vi "Add Menu Items.vi"(7 "Menu control":enum16{"Pulse", "Post-process", "Monitor"}(ring), 8 "error in (no error)":errorcluster, 9 "Reset":bool, 10 "Item Names":string[](array[string]), 11 "Monitor-Pulse in":refnum<class "Application Controller.lvclass">) -> (0 "error out":errorcluster, 3 "Monitor-Pulse out":refnum<class "Application Controller.lvclass">)   [LabVIEW 2016, in "Application Controller.lvclass"]
uses:
  Application Controller.lvclass
  Application Controller.lvclass/Application Controller.ctl
  Read Monitor ref.vi
  Write Monitor ref.vi
  Read Postproc ref.vi
  Write Postproc ref.vi
  NHMFL_Core/Libraries/Queued Listbox/Queued Listbox.xctl
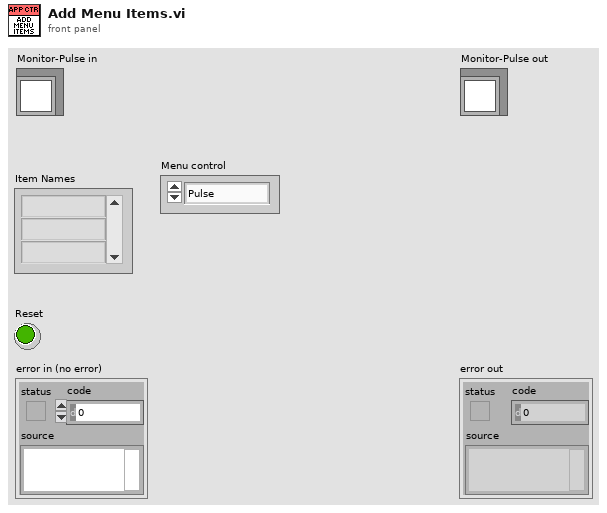
[diagram p1: front panel]
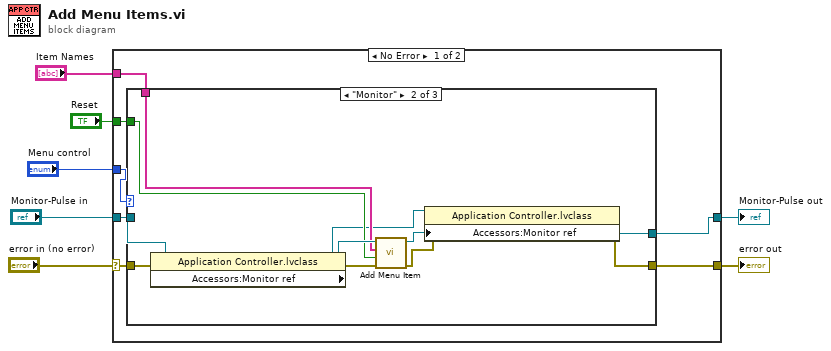
[diagram p0: block diagram]
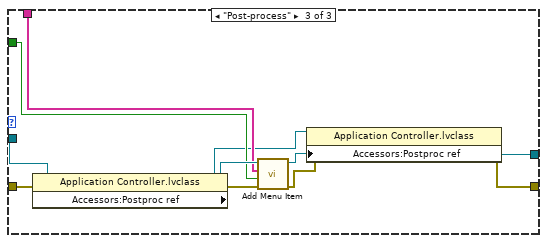
[diagram p3: hidden frame]
diagram:
  n1 = case shown="No Error" "error in (no error)" {
    selector: "error in (no error)" -> [w10 w40]
    tunnel: [w9 w40] -> w6
    tunnel: [w14 w39] -> w4
    tunnel: "Monitor-Pulse in" -> [w11 w39]
    tunnel: "Item Names" -> [w13 _]
    tunnel: "Reset" -> [w12 _]
    tunnel: "Menu control" -> [w8 _]
    frame No Error {
      n2 = case shown="\"Monitor\"" w8 {
        tunnel: [w16 w25 w36] -> w14
        tunnel: w13 -> [_ w24 w35]
        tunnel: w12 -> [_ w23 w34]
        tunnel: w11 -> [w16 w22 w33]
        tunnel: w10 -> [w15 w19 w30]
        tunnel: [w15 w18 w29] -> w9
        frame "Pulse", Default {
        }
        frame "Monitor" {
          n3 = property class="Application Controller.lvclass"(reference=w22, error in=w19) -> (reference out=w21:refnum<class "Application Controller.lvclass">, error out=w20:errorcluster, "Accessors:Monitor ref"=w27:refnum<vi>)
          n4 = call "Add Menu Item.vi"("error in (no error)"=w20, "Reset"=w23, "Item Names"=w24, "Queed Listbox ref"=w27) -> ("error out"=w17:errorcluster, "Queed Listbox ref out"=w26:refnum<vi>)  [unwired: 5 in, 1 out]
          n5 = property class="Application Controller.lvclass"(reference=w21, error in=w17, "Accessors:Monitor ref"=w26) -> (reference out=w25:refnum<class "Application Controller.lvclass">, error out=w18:errorcluster)
        }
        frame "Post-process" {
          n6 = property class="Application Controller.lvclass"(reference=w33, error in=w30) -> (reference out=w32:refnum<class "Application Controller.lvclass">, error out=w31:errorcluster, "Accessors:Postproc ref"=w38:refnum<vi>)
          n7 = call "Add Menu Item.vi"("error in (no error)"=w31, "Reset"=w34, "Item Names"=w35, "Queed Listbox ref"=w38) -> ("error out"=w28:errorcluster, "Queed Listbox ref out"=w37:refnum<vi>)  [unwired: 5 in, 1 out]
          n8 = property class="Application Controller.lvclass"(reference=w32, error in=w28, "Accessors:Postproc ref"=w37) -> (reference out=w36:refnum<class "Application Controller.lvclass">, error out=w29:errorcluster)
        }
      }
    }
    frame Error {
    }
  }
  "error out" <- w6
  "Monitor-Pulse out" <- w4
